vi "NI9252_DataCollection.vi"() -> ()   [LabVIEW 2022 SP3]
panel:
  out "Waveform Chart 4":dynamicdata(graph)
  out "Waveform Chart 3":dynamicdata(graph)
  out "Waveform Chart 2":dynamicdata(graph)
  out "Waveform Chart":dynamicdata(graph)
  in  "stop (F)":bool
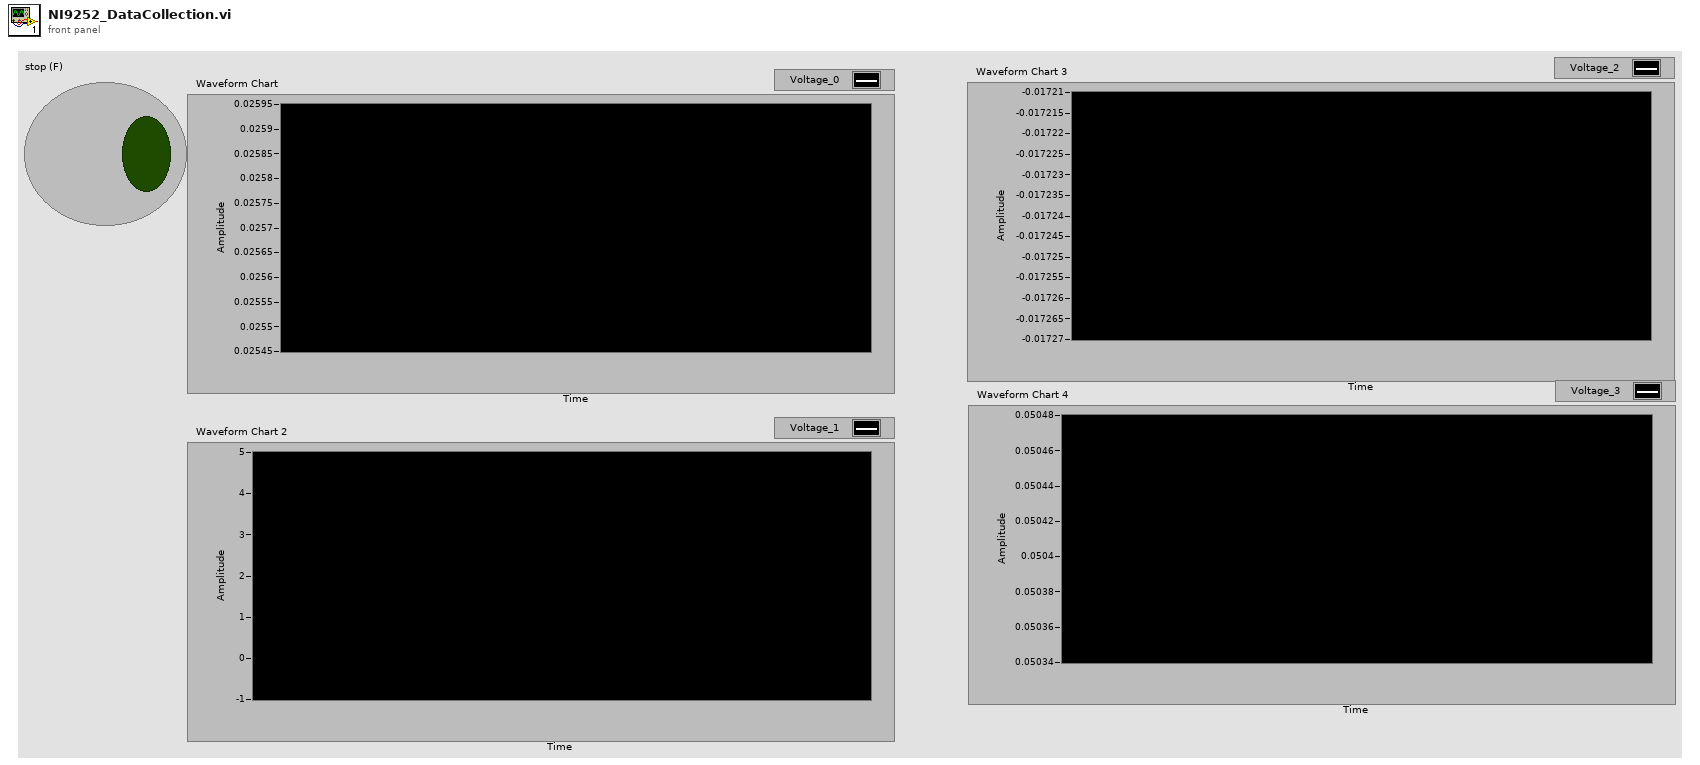
[diagram p1: front panel]
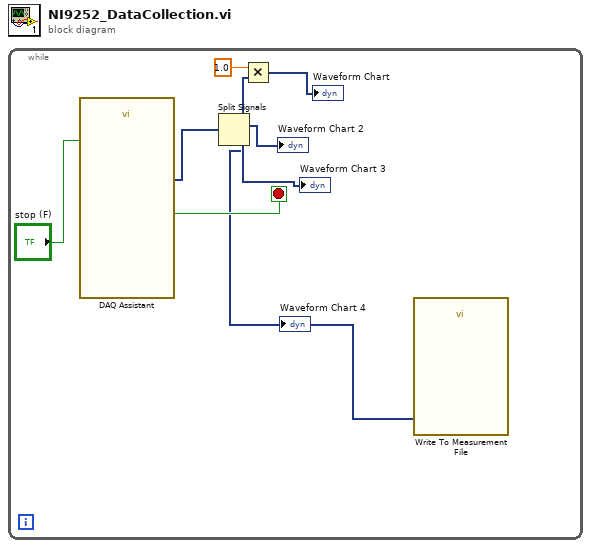
[diagram p0: block diagram]
diagram:
  n1 = while {
    stop <- w8 stop-if-true
    n2 = call "DAQ Assistant"("stop (F)"="stop (F)") -> ("data"=w7:dynamicdata, "stopped"=w8:bool)  [unwired: 15 in, 2 out]
    n3 = Split Signals(w7) -> (w2:dynamicdata, →"Waveform Chart 2":dynamicdata, →"Waveform Chart 3":dynamicdata, w1:dynamicdata)  [unwired: 4 in]
    "Waveform Chart 4" <- w1
    n4 = Multiply(x=1.0, y=w2) -> (x*y=→"Waveform Chart":dynamicdata)
    n5 = call "Write To Measurement File"("Signals"=w1) -> ()  [unwired: 16 in, 3 out]
  }
